vi "CSTK_Button_Icon_Init.vi"(3 "Container State":T20 caption="容器状态", 4 "Previous State":variant caption="前期状态", 5 "Previous Version":T19 caption="前期版本") -> (2 "Current State":T1={"ButtonSize"={"False"={"Width"=0, "Height"=0}, "True"={"Width"=0, "Height"=0}, "True to False"={"Width"=0, "Height"=0}, "False to True"={"Width"=0, "Height"=0}, "Hover in False"={"Width"=0, "Height"=0}, "Hover in True"={"Width"=0, "Height"=0}}, "Logo Image"={"False"={"image type"=0, "image depth"=0, "image"=[], "mask"=[], "colors"=[], "Rectangle"={"left"=0, "top"=0, "right"=0, "bottom"=0}}, "True"={"image type"=0, "image depth"=0, "image"=[], "mask"=[], "colors"=[], "Rectangle"={"left"=0, "top"=0, "right"=0, "bottom"=0}}, "True to False"={"image type"=0, "image depth"=0, "image"=[], "mask"=[], "colors"=[], "Rectangle"={"left"=0, "top"=0, "right"=0, "bottom"=0}}, "False to True"={"image type"=0, "image depth"=0, "image"=[], "mask"=[], "colors"=[], "Rectangle"={"left"=0, "top"=0, "right"=0, "bottom"=0}}, "Hover in False"={"image type"=0, "image depth"=0, "image"=[], "mask"=[], "colors"=[], "Rectangle"={"left"=0, "top"=0, "right"=0, "bottom"=0}}, "Hover in True"={"image type"=0, "image depth"=0, "image"=[], "mask"=[], "colors"=[], "Rectangle"={"left"=0, "top"=0, "right"=0, "bottom"=0}}}, "Logo Properties"={"False"={"Display Logo?"=FALSE, "Horizontal Offset"=0}, "True"={"Display Logo?"=FALSE, "Horizontal Offset"=0}, "True to False"={"Display Logo?"=FALSE, "Horizontal Offset"=0}, "False to True"={"Display Logo?"=FALSE, "Horizontal Offset"=0}, "Hover in False"={"Display Logo?"=FALSE, "Horizontal Offset"=0}, "Hover in True"={"Display Logo?"=FALSE, "Horizontal Offset"=0}}, "Text String"={"False"="", "True"="", "True to False"="", "False to True"="", "Hover in False"="", "Hover in True"=""}, "Text Properties"={"False"={"Display Text?"=FALSE, "Text Color"=0, "Horizontal Offset"=0, "Font Style"={"Font Name"="", "Size"=0, "Strikeout?"=FALSE, "Italic?"=FALSE, "Underline?"=FALSE, "Outline?"=FALSE, "Shadow?"=FALSE, "Bold?"=FALSE}}, "True"={"Display Text?"=FALSE, "Text Color"=0, "Horizontal Offset"=0, "Font Style"={"Font Name"="", "Size"=0, "Strikeout?"=FALSE, "Italic?"=FALSE, "Underline?"=FALSE, "Outline?"=FALSE, "Shadow?"=FALSE, "Bold?"=FALSE}}, "True to False"={"Display Text?"=FALSE, "Text Color"=0, "Horizontal Offset"=0, "Font Style"={"Font Name"="", "Size"=0, "Strikeout?"=FALSE, "Italic?"=FALSE, "Underline?"=FALSE, "Outline?"=FALSE, "Shadow?"=FALSE, "Bold?"=FALSE}}, "False to True"={"Display Text?"=FALSE, "Text Color"=0, "Horizontal Offset"=0, "Font Style"={"Font Name"="", "Size"=0, "Strikeout?"=FALSE, "Italic?"=FALSE, "Underline?"=FALSE, "Outline?"=FALSE, "Shadow?"=FALSE, "Bold?"=FALSE}}, "Hover in False"={"Display Text?"=FALSE, "Text Color"=0, "Horizontal Offset"=0, "Font Style"={"Font Name"="", "Size"=0, "Strikeout?"=FALSE, "Italic?"=FALSE, "Underline?"=FALSE, "Outline?"=FALSE, "Shadow?"=FALSE, "Bold?"=FALSE}}, "Hover in True"={"Display Text?"=FALSE, "Text Color"=0, "Horizontal Offset"=0, "Font Style"={"Font Name"="", "Size"=0, "Strikeout?"=FALSE, "Italic?"=FALSE, "Underline?"=FALSE, "Outline?"=FALSE, "Shadow?"=FALSE, "Bold?"=FALSE}}}, "BG Color"={"False"=0, "True"=0, "True to False"=0, "False to True"=0, "Hover in False"=0, "Hover in True"=0}, "Border Color"={"False"=0, "True"=0, "True to False"=0, "False to True"=0, "Hover in False"=0, "Hover in True"=0}, "Border Properties"={"False"={"Radius"=0, "Border Style"={"Width"=3, "Style"=enum."Solid"}}, "True"={"Radius"=0, "Border Style"={"Width"=3, "Style"=enum."Solid"}}, "True to False"={"Radius"=0, "Border Style"={"Width"=3, "Style"=enum."Solid"}}, "False to True"={"Radius"=0, "Border Style"={"Width"=3, "Style"=enum."Solid"}}, "Hover in False"={"Radius"=0, "Border Style"={"Width"=3, "Style"=enum."Solid"}}, "Hover in True"={"Radius"=0, "Border Style"={"Width"=3, "Style"=enum."Solid"}}}, "Current BG Image"={"False"=bytes[0], "True"=bytes[0], "True to False"=bytes[0], "False to True"=bytes[0], "Hover in False"=bytes[0], "Hover in True"=bytes[0]}, "DrawAreaSize"={"False"={"Width"=0, "Height"=0}, "True"={"Width"=0, "Height"=0}, "True to False"={"Width"=0, "Height"=0}, "False to True"={"Width"=0, "Height"=0}, "Hover in False"={"Width"=0, "Height"=0}, "Hover in True"={"Width"=0, "Height"=0}}, "Text String Offset"={"False"=0, "True"=0, "True to False"=0, "False to True"=0, "Hover in False"=0, "Hover in True"=0}} caption="当前状态")   [LabVIEW 2015, in "CSTK_Button_Icon.xctl"]
uses:
  CSTK_Button_Icon.xctl
  CSTK_Button_Icon_Status.ctl
  Private/TypeDefinitions/_CSTK_Button_Icon_ButtonSize.ctl
  <vilib>/Utility/miscctls.llb/LVBoundsTypeDef.ctl
  Private/TypeDefinitions/_CSTK_Button_Icon_LogoImage.ctl
  <vilib>/picture/picture.llb/imagedata.ctl
  Private/TypeDefinitions/_CSTK_Button_Icon_LogoProperties.ctl
  Private/TypeDefinitions/_CSTK_Button_Icon_LogoProperties_Data.ctl
  Private/TypeDefinitions/_CSTK_Button_Icon_TextString.ctl
  Private/TypeDefinitions/_CSTK_Button_Icon_TextProperties.ctl
  Private/TypeDefinitions/_CSTK_Button_Icon_TextProperties_Data.ctl
  Private/TypeDefinitions/_CSTK_Button_Icon_TextProperties_FontStyle.ctl
  Private/TypeDefinitions/_CSTK_Button_Icon_BGColor.ctl
  Private/TypeDefinitions/_CSTK_Button_Icon_BorderColor.ctl
  Private/TypeDefinitions/_CSTK_Button_Icon_BorderProperties.ctl
  Private/TypeDefinitions/_CSTK_Button_Icon_BorderProperties_Data.ctl
  Private/TypeDefinitions/_CSTK_Button_Icon_CurrentBGImage.ctl
  Private/TypeDefinitions/_CSTK_Button_Icon_DrawAreaSize.ctl
  Private/TypeDefinitions/_CSTK_Button_Icon_TextStartOffset.ctl
  <vilib>/_xctls/Container State.ctl
  <vilib>/_xctls/Version.ctl
  <vilib>/_xctls/XControlSupport.lvlib
panel:
  in  "Default Indicator State":T1={"ButtonSize"={"False"={"Width"=120, "Height"=36}, "True"={"Width"=120, "Height"=36}, "True to False"={"Width"=120, "Height"=36}, "False to True"={"Width"=120, "Height"=36}, "Hover in False"={"Width"=120, "Height"=36}, "Hover in True"={"Width"=120, "Height"=36}}, "Logo Image"={"False"={"image type"=0, "image depth"=32, "image"=array[2304 elements], "mask"=[0, 0, 0, 0, 0, 0, 0, 0, 0, 0, 0, 0, 0, 0, 0, 0, 0, 0, 0, 0, 0, 0, 12, 0, 0, 0, 28, 0, 0, 0, 60, 0, 0, 0, 120, 0, 0, 0, 240, 0, 48, 1, 224, 0, 56, 3, 192, 0, 28, 7, 128, 0, 14, 15, 0, 0, 7, 30, 0, 0, 3, 188, 0, 0, 1, 248, 0, 0, 0, 240, 0, 0, 0, 96, 0, 0, 0, 0, 0, 0, 0, 0, 0, 0, 0, 0, 0, 0, 0, 0, 0, 0, 0, 0, 0, 0], "colors"=[], "Rectangle"={"left"=0, "top"=0, "right"=24, "bottom"=24}}, "True"={"image type"=0, "image depth"=32, "image"=array[2304 elements], "mask"=[0, 0, 0, 0, 0, 0, 0, 0, 0, 0, 0, 0, 0, 0, 0, 0, 0, 0, 0, 0, 0, 0, 12, 0, 0, 0, 28, 0, 0, 0, 60, 0, 0, 0, 120, 0, 0, 0, 240, 0, 48, 1, 224, 0, 56, 3, 192, 0, 28, 7, 128, 0, 14, 15, 0, 0, 7, 30, 0, 0, 3, 188, 0, 0, 1, 248, 0, 0, 0, 240, 0, 0, 0, 96, 0, 0, 0, 0, 0, 0, 0, 0, 0, 0, 0, 0, 0, 0, 0, 0, 0, 0, 0, 0, 0, 0], "colors"=[], "Rectangle"={"left"=0, "top"=0, "right"=24, "bottom"=24}}, "True to False"={"image type"=0, "image depth"=32, "image"=array[2304 elements], "mask"=[0, 0, 0, 0, 0, 0, 0, 0, 0, 0, 0, 0, 0, 0, 0, 0, 0, 0, 0, 0, 0, 0, 12, 0, 0, 0, 28, 0, 0, 0, 60, 0, 0, 0, 120, 0, 0, 0, 240, 0, 48, 1, 224, 0, 56, 3, 192, 0, 28, 7, 128, 0, 14, 15, 0, 0, 7, 30, 0, 0, 3, 188, 0, 0, 1, 248, 0, 0, 0, 240, 0, 0, 0, 96, 0, 0, 0, 0, 0, 0, 0, 0, 0, 0, 0, 0, 0, 0, 0, 0, 0, 0, 0, 0, 0, 0], "colors"=[], "Rectangle"={"left"=0, "top"=0, "right"=24, "bottom"=24}}, "False to True"={"image type"=0, "image depth"=32, "image"=array[2304 elements], "mask"=[0, 0, 0, 0, 0, 0, 0, 0, 0, 0, 0, 0, 0, 0, 0, 0, 0, 0, 0, 0, 0, 0, 12, 0, 0, 0, 28, 0, 0, 0, 60, 0, 0, 0, 120, 0, 0, 0, 240, 0, 48, 1, 224, 0, 56, 3, 192, 0, 28, 7, 128, 0, 14, 15, 0, 0, 7, 30, 0, 0, 3, 188, 0, 0, 1, 248, 0, 0, 0, 240, 0, 0, 0, 96, 0, 0, 0, 0, 0, 0, 0, 0, 0, 0, 0, 0, 0, 0, 0, 0, 0, 0, 0, 0, 0, 0], "colors"=[], "Rectangle"={"left"=0, "top"=0, "right"=24, "bottom"=24}}, "Hover in False"={"image type"=0, "image depth"=32, "image"=array[2304 elements], "mask"=[0, 0, 0, 0, 0, 0, 0, 0, 0, 0, 0, 0, 0, 0, 0, 0, 0, 0, 0, 0, 0, 0, 12, 0, 0, 0, 28, 0, 0, 0, 60, 0, 0, 0, 120, 0, 0, 0, 240, 0, 48, 1, 224, 0, 56, 3, 192, 0, 28, 7, 128, 0, 14, 15, 0, 0, 7, 30, 0, 0, 3, 188, 0, 0, 1, 248, 0, 0, 0, 240, 0, 0, 0, 96, 0, 0, 0, 0, 0, 0, 0, 0, 0, 0, 0, 0, 0, 0, 0, 0, 0, 0, 0, 0, 0, 0], "colors"=[], "Rectangle"={"left"=0, "top"=0, "right"=24, "bottom"=24}}, "Hover in True"={"image type"=0, "image depth"=32, "image"=array[2304 elements], "mask"=[0, 0, 0, 0, 0, 0, 0, 0, 0, 0, 0, 0, 0, 0, 0, 0, 0, 0, 0, 0, 0, 0, 12, 0, 0, 0, 28, 0, 0, 0, 60, 0, 0, 0, 120, 0, 0, 0, 240, 0, 48, 1, 224, 0, 56, 3, 192, 0, 28, 7, 128, 0, 14, 15, 0, 0, 7, 30, 0, 0, 3, 188, 0, 0, 1, 248, 0, 0, 0, 240, 0, 0, 0, 96, 0, 0, 0, 0, 0, 0, 0, 0, 0, 0, 0, 0, 0, 0, 0, 0, 0, 0, 0, 0, 0, 0], "colors"=[], "Rectangle"={"left"=0, "top"=0, "right"=24, "bottom"=24}}}, "Logo Properties"={"False"={"Display Logo?"=TRUE, "Horizontal Offset"=0}, "True"={"Display Logo?"=TRUE, "Horizontal Offset"=0}, "True to False"={"Display Logo?"=TRUE, "Horizontal Offset"=0}, "False to True"={"Display Logo?"=TRUE, "Horizontal Offset"=0}, "Hover in False"={"Display Logo?"=TRUE, "Horizontal Offset"=0}, "Hover in True"={"Display Logo?"=TRUE, "Horizontal Offset"=0}}, "Text String"={"False"="Fasle", "True"="True", "True to False"="False", "False to True"="True", "Hover in False"="Fasle", "Hover in True"="True"}, "Text Properties"={"False"={"Display Text?"=TRUE, "Text Color"=0, "Horizontal Offset"=0, "Font Style"={"Font Name"="", "Size"=17, "Strikeout?"=FALSE, "Italic?"=FALSE, "Underline?"=FALSE, "Outline?"=FALSE, "Shadow?"=FALSE, "Bold?"=FALSE}}, "True"={"Display Text?"=TRUE, "Text Color"=0, "Horizontal Offset"=0, "Font Style"={"Font Name"="", "Size"=17, "Strikeout?"=FALSE, "Italic?"=FALSE, "Underline?"=FALSE, "Outline?"=FALSE, "Shadow?"=FALSE, "Bold?"=FALSE}}, "True to False"={"Display Text?"=TRUE, "Text Color"=0, "Horizontal Offset"=0, "Font Style"={"Font Name"="", "Size"=17, "Strikeout?"=FALSE, "Italic?"=FALSE, "Underline?"=FALSE, "Outline?"=FALSE, "Shadow?"=FALSE, "Bold?"=FALSE}}, "False to True"={"Display Text?"=TRUE, "Text Color"=0, "Horizontal Offset"=0, "Font Style"={"Font Name"="", "Size"=17, "Strikeout?"=FALSE, "Italic?"=FALSE, "Underline?"=FALSE, "Outline?"=FALSE, "Shadow?"=FALSE, "Bold?"=FALSE}}, "Hover in False"={"Display Text?"=TRUE, "Text Color"=0, "Horizontal Offset"=0, "Font Style"={"Font Name"="", "Size"=17, "Strikeout?"=FALSE, "Italic?"=FALSE, "Underline?"=FALSE, "Outline?"=FALSE, "Shadow?"=FALSE, "Bold?"=FALSE}}, "Hover in True"={"Display Text?"=TRUE, "Text Color"=0, "Horizontal Offset"=0, "Font Style"={"Font Name"="", "Size"=17, "Strikeout?"=FALSE, "Italic?"=FALSE, "Underline?"=FALSE, "Outline?"=FALSE, "Shadow?"=FALSE, "Bold?"=FALSE}}}, "BG Color"={"False"=14869218, "True"=16744576, "True to False"=14869218, "False to True"=16744576, "Hover in False"=14869218, "Hover in True"=16744576}, "Border Color"={"False"=11251123, "True"=11251123, "True to False"=11251123, "False to True"=11251123, "Hover in False"=11251123, "Hover in True"=11251123}, "Border Properties"={"False"={"Radius"=10, "Border Style"={"Width"=3, "Style"=enum."Solid"}}, "True"={"Radius"=10, "Border Style"={"Width"=3, "Style"=enum."Solid"}}, "True to False"={"Radius"=10, "Border Style"={"Width"=3, "Style"=enum."Solid"}}, "False to True"={"Radius"=10, "Border Style"={"Width"=3, "Style"=enum."Solid"}}, "Hover in False"={"Radius"=10, "Border Style"={"Width"=3, "Style"=enum."Solid"}}, "Hover in True"={"Radius"=10, "Border Style"={"Width"=3, "Style"=enum."Solid"}}}, "Current BG Image"={"False"=bytes[0], "True"=bytes[0], "True to False"=bytes[0], "False to True"=bytes[0], "Hover in False"=bytes[0], "Hover in True"=bytes[0]}, "DrawAreaSize"={"False"={"Width"=0, "Height"=0}, "True"={"Width"=0, "Height"=0}, "True to False"={"Width"=0, "Height"=0}, "False to True"={"Width"=0, "Height"=0}, "Hover in False"={"Width"=0, "Height"=0}, "Hover in True"={"Width"=0, "Height"=0}}, "Text String Offset"={"False"=0, "True"=0, "True to False"=0, "False to True"=0, "Hover in False"=0, "Hover in True"=0}} caption="默认显示控件状态"
  in  "Default Control State":T1={"ButtonSize"={"False"={"Width"=120, "Height"=36}, "True"={"Width"=120, "Height"=36}, "True to False"={"Width"=120, "Height"=36}, "False to True"={"Width"=120, "Height"=36}, "Hover in False"={"Width"=120, "Height"=36}, "Hover in True"={"Width"=120, "Height"=36}}, "Logo Image"={"False"={"image type"=0, "image depth"=32, "image"=array[2304 elements], "mask"=[0, 0, 0, 0, 0, 0, 0, 0, 0, 0, 0, 0, 0, 0, 0, 0, 0, 0, 0, 0, 0, 0, 12, 0, 0, 0, 28, 0, 0, 0, 60, 0, 0, 0, 120, 0, 0, 0, 240, 0, 48, 1, 224, 0, 56, 3, 192, 0, 28, 7, 128, 0, 14, 15, 0, 0, 7, 30, 0, 0, 3, 188, 0, 0, 1, 248, 0, 0, 0, 240, 0, 0, 0, 96, 0, 0, 0, 0, 0, 0, 0, 0, 0, 0, 0, 0, 0, 0, 0, 0, 0, 0, 0, 0, 0, 0], "colors"=[], "Rectangle"={"left"=0, "top"=0, "right"=24, "bottom"=24}}, "True"={"image type"=0, "image depth"=32, "image"=array[2304 elements], "mask"=[0, 0, 0, 0, 0, 0, 0, 0, 0, 0, 0, 0, 0, 0, 0, 0, 0, 0, 0, 0, 0, 0, 12, 0, 0, 0, 28, 0, 0, 0, 60, 0, 0, 0, 120, 0, 0, 0, 240, 0, 48, 1, 224, 0, 56, 3, 192, 0, 28, 7, 128, 0, 14, 15, 0, 0, 7, 30, 0, 0, 3, 188, 0, 0, 1, 248, 0, 0, 0, 240, 0, 0, 0, 96, 0, 0, 0, 0, 0, 0, 0, 0, 0, 0, 0, 0, 0, 0, 0, 0, 0, 0, 0, 0, 0, 0], "colors"=[], "Rectangle"={"left"=0, "top"=0, "right"=24, "bottom"=24}}, "True to False"={"image type"=0, "image depth"=32, "image"=array[2304 elements], "mask"=[0, 0, 0, 0, 0, 0, 0, 0, 0, 0, 0, 0, 0, 0, 0, 0, 0, 0, 0, 0, 0, 0, 12, 0, 0, 0, 28, 0, 0, 0, 60, 0, 0, 0, 120, 0, 0, 0, 240, 0, 48, 1, 224, 0, 56, 3, 192, 0, 28, 7, 128, 0, 14, 15, 0, 0, 7, 30, 0, 0, 3, 188, 0, 0, 1, 248, 0, 0, 0, 240, 0, 0, 0, 96, 0, 0, 0, 0, 0, 0, 0, 0, 0, 0, 0, 0, 0, 0, 0, 0, 0, 0, 0, 0, 0, 0], "colors"=[], "Rectangle"={"left"=0, "top"=0, "right"=24, "bottom"=24}}, "False to True"={"image type"=0, "image depth"=32, "image"=array[2304 elements], "mask"=[0, 0, 0, 0, 0, 0, 0, 0, 0, 0, 0, 0, 0, 0, 0, 0, 0, 0, 0, 0, 0, 0, 12, 0, 0, 0, 28, 0, 0, 0, 60, 0, 0, 0, 120, 0, 0, 0, 240, 0, 48, 1, 224, 0, 56, 3, 192, 0, 28, 7, 128, 0, 14, 15, 0, 0, 7, 30, 0, 0, 3, 188, 0, 0, 1, 248, 0, 0, 0, 240, 0, 0, 0, 96, 0, 0, 0, 0, 0, 0, 0, 0, 0, 0, 0, 0, 0, 0, 0, 0, 0, 0, 0, 0, 0, 0], "colors"=[], "Rectangle"={"left"=0, "top"=0, "right"=24, "bottom"=24}}, "Hover in False"={"image type"=0, "image depth"=32, "image"=array[2304 elements], "mask"=[0, 0, 0, 0, 0, 0, 0, 0, 0, 0, 0, 0, 0, 0, 0, 0, 0, 0, 0, 0, 0, 0, 12, 0, 0, 0, 28, 0, 0, 0, 60, 0, 0, 0, 120, 0, 0, 0, 240, 0, 48, 1, 224, 0, 56, 3, 192, 0, 28, 7, 128, 0, 14, 15, 0, 0, 7, 30, 0, 0, 3, 188, 0, 0, 1, 248, 0, 0, 0, 240, 0, 0, 0, 96, 0, 0, 0, 0, 0, 0, 0, 0, 0, 0, 0, 0, 0, 0, 0, 0, 0, 0, 0, 0, 0, 0], "colors"=[], "Rectangle"={"left"=0, "top"=0, "right"=24, "bottom"=24}}, "Hover in True"={"image type"=0, "image depth"=32, "image"=array[2304 elements], "mask"=[0, 0, 0, 0, 0, 0, 0, 0, 0, 0, 0, 0, 0, 0, 0, 0, 0, 0, 0, 0, 0, 0, 12, 0, 0, 0, 28, 0, 0, 0, 60, 0, 0, 0, 120, 0, 0, 0, 240, 0, 48, 1, 224, 0, 56, 3, 192, 0, 28, 7, 128, 0, 14, 15, 0, 0, 7, 30, 0, 0, 3, 188, 0, 0, 1, 248, 0, 0, 0, 240, 0, 0, 0, 96, 0, 0, 0, 0, 0, 0, 0, 0, 0, 0, 0, 0, 0, 0, 0, 0, 0, 0, 0, 0, 0, 0], "colors"=[], "Rectangle"={"left"=0, "top"=0, "right"=24, "bottom"=24}}}, "Logo Properties"={"False"={"Display Logo?"=TRUE, "Horizontal Offset"=0}, "True"={"Display Logo?"=TRUE, "Horizontal Offset"=0}, "True to False"={"Display Logo?"=TRUE, "Horizontal Offset"=0}, "False to True"={"Display Logo?"=TRUE, "Horizontal Offset"=0}, "Hover in False"={"Display Logo?"=TRUE, "Horizontal Offset"=0}, "Hover in True"={"Display Logo?"=TRUE, "Horizontal Offset"=0}}, "Text String"={"False"="OK", "True"="OK", "True to False"="OK", "False to True"="OK", "Hover in False"="OK", "Hover in True"="OK"}, "Text Properties"={"False"={"Display Text?"=TRUE, "Text Color"=0, "Horizontal Offset"=0, "Font Style"={"Font Name"="", "Size"=17, "Strikeout?"=FALSE, "Italic?"=FALSE, "Underline?"=FALSE, "Outline?"=FALSE, "Shadow?"=FALSE, "Bold?"=FALSE}}, "True"={"Display Text?"=TRUE, "Text Color"=0, "Horizontal Offset"=0, "Font Style"={"Font Name"="", "Size"=17, "Strikeout?"=FALSE, "Italic?"=FALSE, "Underline?"=FALSE, "Outline?"=FALSE, "Shadow?"=FALSE, "Bold?"=FALSE}}, "True to False"={"Display Text?"=TRUE, "Text Color"=0, "Horizontal Offset"=0, "Font Style"={"Font Name"="", "Size"=17, "Strikeout?"=FALSE, "Italic?"=FALSE, "Underline?"=FALSE, "Outline?"=FALSE, "Shadow?"=FALSE, "Bold?"=FALSE}}, "False to True"={"Display Text?"=TRUE, "Text Color"=0, "Horizontal Offset"=0, "Font Style"={"Font Name"="", "Size"=17, "Strikeout?"=FALSE, "Italic?"=FALSE, "Underline?"=FALSE, "Outline?"=FALSE, "Shadow?"=FALSE, "Bold?"=FALSE}}, "Hover in False"={"Display Text?"=TRUE, "Text Color"=0, "Horizontal Offset"=0, "Font Style"={"Font Name"="", "Size"=17, "Strikeout?"=FALSE, "Italic?"=FALSE, "Underline?"=FALSE, "Outline?"=FALSE, "Shadow?"=FALSE, "Bold?"=FALSE}}, "Hover in True"={"Display Text?"=TRUE, "Text Color"=0, "Horizontal Offset"=0, "Font Style"={"Font Name"="", "Size"=17, "Strikeout?"=FALSE, "Italic?"=FALSE, "Underline?"=FALSE, "Outline?"=FALSE, "Shadow?"=FALSE, "Bold?"=FALSE}}}, "BG Color"={"False"=12632319, "True"=16761024, "True to False"=8421631, "False to True"=16744576, "Hover in False"=10263807, "Hover in True"=16751772}, "Border Color"={"False"=11251123, "True"=11251123, "True to False"=11251123, "False to True"=11251123, "Hover in False"=11251123, "Hover in True"=11251123}, "Border Properties"={"False"={"Radius"=10, "Border Style"={"Width"=3, "Style"=enum."Solid"}}, "True"={"Radius"=10, "Border Style"={"Width"=3, "Style"=enum."Solid"}}, "True to False"={"Radius"=10, "Border Style"={"Width"=3, "Style"=enum."Solid"}}, "False to True"={"Radius"=10, "Border Style"={"Width"=3, "Style"=enum."Solid"}}, "Hover in False"={"Radius"=10, "Border Style"={"Width"=3, "Style"=enum."Solid"}}, "Hover in True"={"Radius"=10, "Border Style"={"Width"=3, "Style"=enum."Solid"}}}, "Current BG Image"={"False"=bytes[0], "True"=bytes[0], "True to False"=bytes[0], "False to True"=bytes[0], "Hover in False"=bytes[0], "Hover in True"=bytes[0]}, "DrawAreaSize"={"False"={"Width"=0, "Height"=0}, "True"={"Width"=0, "Height"=0}, "True to False"={"Width"=0, "Height"=0}, "False to True"={"Width"=0, "Height"=0}, "Hover in False"={"Width"=0, "Height"=0}, "Hover in True"={"Width"=0, "Height"=0}}, "Text String Offset"={"False"=0, "True"=0, "True to False"=0, "False to True"=0, "Hover in False"=0, "Hover in True"=0}} caption="默认输入控件状态"
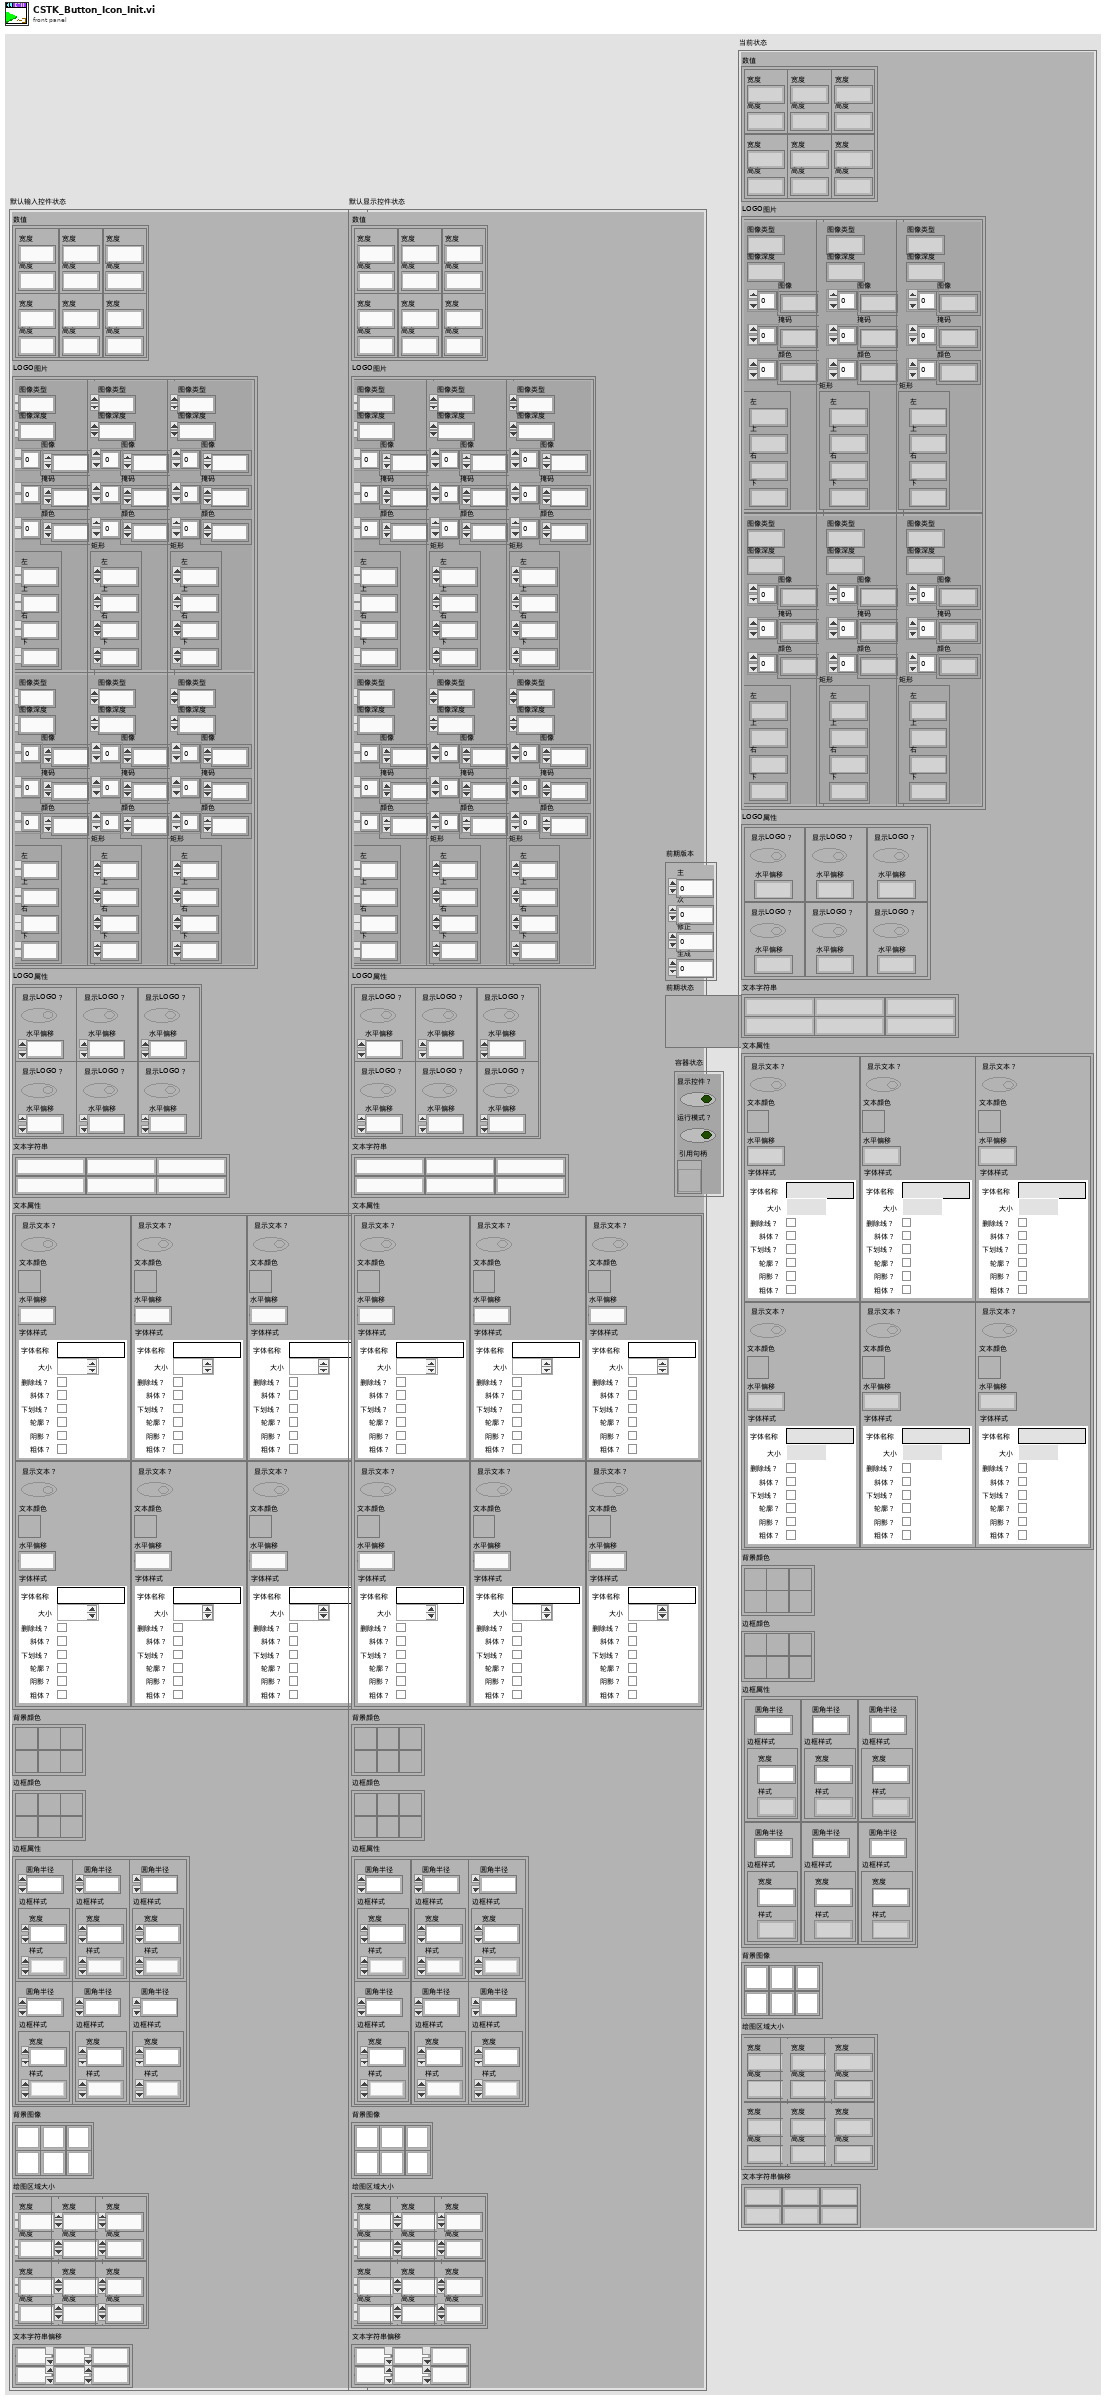
[diagram p1: front panel]
types:
  T1 = typedef "CSTK_Button_Icon.xctl/CSTK_Button_Icon_Status.ctl" = cluster{"ButtonSize":T2, "Logo Image":T4, "Logo Properties":T6, "Text String":T8, "Text Properties":T9, "BG Color":T12, "Border Color":T13, "Border Properties":T14, "Current BG Image":T16, "DrawAreaSize":T17, "Text String Offset":T18}
  T2 = typedef "CSTK_Button_Icon.xctl/_CSTK_Button_Icon_ButtonSize.ctl" = cluster{"False":T3, "True":T3, "True to False":T3, "False to True":T3, "Hover in False":T3, "Hover in True":T3}
  T3 = typedef "LVBoundsTypeDef.ctl" = cluster{"Width":u32, "Height":u32}
  T4 = typedef "CSTK_Button_Icon.xctl/_CSTK_Button_Icon_LogoImage.ctl" = cluster{"False":T5, "True":T5, "True to False":T5, "False to True":T5, "Hover in False":T5, "Hover in True":T5}
  T5 = typedef "imagedata.ctl" = cluster{"image type":i32, "image depth":i32, "image":u8[], "mask":u8[], "colors":u32[], "Rectangle":cluster{"left":i16, "top":i16, "right":i16, "bottom":i16}}
  T6 = typedef "CSTK_Button_Icon.xctl/_CSTK_Button_Icon_LogoProperties.ctl" = cluster{"False":T7, "True":T7, "True to False":T7, "False to True":T7, "Hover in False":T7, "Hover in True":T7}
  T7 = typedef "CSTK_Button_Icon.xctl/_CSTK_Button_Icon_LogoProperties_Data.ctl" = cluster{"Display Logo?":bool, "Horizontal Offset":i16}
  T8 = typedef "CSTK_Button_Icon.xctl/_CSTK_Button_Icon_TextString.ctl" = cluster{"False":string, "True":string, "True to False":string, "False to True":string, "Hover in False":string, "Hover in True":string}
  T9 = typedef "CSTK_Button_Icon.xctl/_CSTK_Button_Icon_TextProperties.ctl" = cluster{"False":T10, "True":T10, "True to False":T10, "False to True":T10, "Hover in False":T10, "Hover in True":T10}
  T10 = typedef "CSTK_Button_Icon.xctl/_CSTK_Button_Icon_TextProperties_Data.ctl" = cluster{"Display Text?":bool, "Text Color":u32, "Horizontal Offset":i16, "Font Style":T11}
  T11 = typedef "CSTK_Button_Icon.xctl/_CSTK_Button_Icon_TextProperties_FontStyle.ctl" = cluster{"Font Name":string, "Size":i16, "Strikeout?":bool, "Italic?":bool, "Underline?":bool, "Outline?":bool, "Shadow?":bool, "Bold?":bool}
  T12 = typedef "CSTK_Button_Icon.xctl/_CSTK_Button_Icon_BGColor.ctl" = cluster{"False":u32, "True":u32, "True to False":u32, "False to True":u32, "Hover in False":u32, "Hover in True":u32}
  T13 = typedef "CSTK_Button_Icon.xctl/_CSTK_Button_Icon_BorderColor.ctl" = cluster{"False":u32, "True":u32, "True to False":u32, "False to True":u32, "Hover in False":u32, "Hover in True":u32}
  T14 = typedef "CSTK_Button_Icon.xctl/_CSTK_Button_Icon_BorderProperties.ctl" = cluster{"False":T15, "True":T15, "True to False":T15, "False to True":T15, "Hover in False":T15, "Hover in True":T15}
  T15 = typedef "CSTK_Button_Icon.xctl/_CSTK_Button_Icon_BorderProperties_Data.ctl" = cluster{"Radius":i16, "Border Style":cluster{"Width":u16, "Style":enum32{"Solid", "Dash", "Dot", "DashDot", "DashDotDot"}}}
  T16 = typedef "CSTK_Button_Icon.xctl/_CSTK_Button_Icon_CurrentBGImage.ctl" = cluster{"False":picture, "True":picture, "True to False":picture, "False to True":picture, "Hover in False":picture, "Hover in True":picture}
  T17 = typedef "CSTK_Button_Icon.xctl/_CSTK_Button_Icon_DrawAreaSize.ctl" = cluster{"False":T3, "True":T3, "True to False":T3, "False to True":T3, "Hover in False":T3, "Hover in True":T3}
  T18 = typedef "CSTK_Button_Icon.xctl/_CSTK_Button_Icon_TextStartOffset.ctl" = cluster{"False":i32, "True":i32, "True to False":i32, "False to True":i32, "Hover in False":i32, "Hover in True":i32}
  T19 = typedef "XControlSupport.lvlib/Version.ctl" = cluster{"Major":u16, "Minor":u16, "Fix":u16, "Build":u16}
  T20 = typedef "XControlSupport.lvlib/Container State.ctl" = cluster{"Indicator?":bool, "Run Mode?":bool, " Refnum":refnum<vi>}
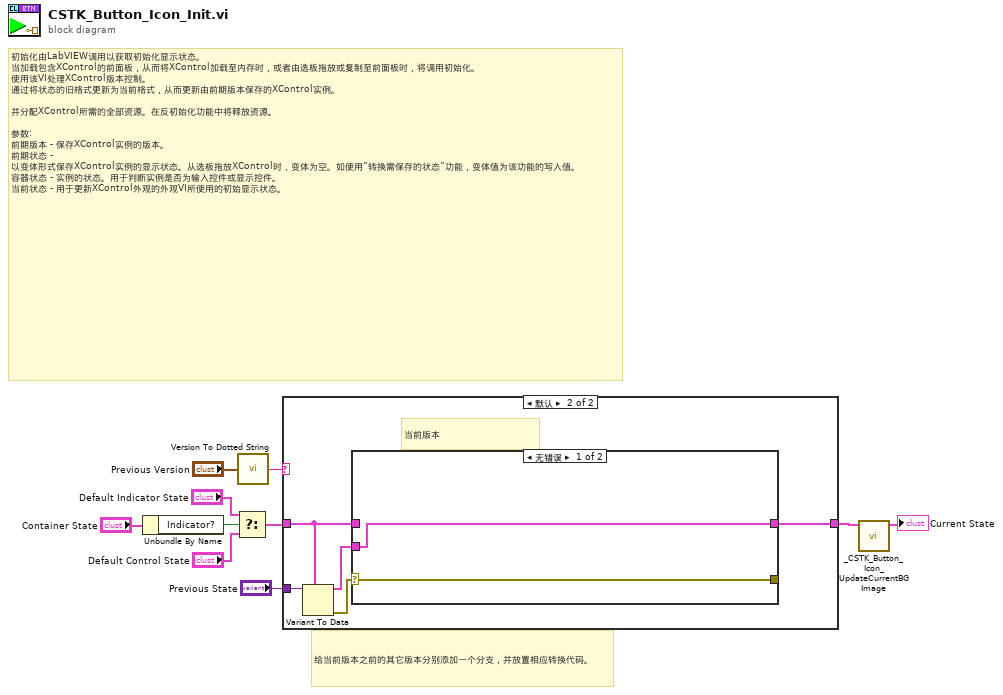
[diagram p0: block diagram]
diagram:
  # "给当前版本之前的其它版本分别添加一个分支，并放置相应转换代码。"
  # "初始化由LabVIEW调用以获取初始化显示状态。\n当加载包含XControl的前面板，从而将XControl加载至内存时，或者由选板拖放或复制至前面板时，将调用初始化。\n使用该VI处理XControl版本控制。\n通过将状态的旧格式更新为当前格式，从而更新由前期版本保存的XControl实例。\n\n并分配XControl所需的全部资源。在反初始化功能中将释放资源。\n\n参数: \n前期版本 - 保存XControl实例的版本。\n前期状态 - 以变体形式保存XControl实例的显示状态。从选板拖放XControl时，变体为空。如使用“转换需保存的状态”功能，变体值为该功能的写入值。\n容器状态 - 实例的状态。用于判断实例是否为输入控件或显示控件。\n当前状态 - 用于更新XControl外观的外观VI所使用的初始显示状态。"
  n1 = Unbundle By Name("Container State") -> ("Indicator?"=w7:bool)
  n2 = Select(t="Default Indicator State", s=w7, f="Default Control State") -> (s? t:f=w6:T1)
  n3 = call <vilib>:"Version To Dotted String.vi"("Version"="Previous Version") -> ("String Version"=w4:string)
  n4 = case shown="默认" w4 {
    tunnel: "Previous State" -> [_ w16]
    tunnel: [w11 w12] -> w2
    tunnel: w6 -> [w11 w13]
    frame "0.0.0.0" {
      # "已创建，并使用默认状态"
    }
    frame Default {
      # "当前版本"
      n5 = Variant To Data(type=w13, Variant=w16) -> (data=w14:T1, error out=w15:errorcluster)  [unwired: 1 in]
      n6 = case shown="无错误" w15 {
        selector: w15 -> [w18 w19]
        tunnel: w14 -> [w17 _]
        tunnel: [w17 w20] -> w12
        tunnel: w13 -> [_ w20]
        tunnel: [w18 w19] -> _
        frame No Error {
        }
        frame Error {
          # "转换前期保存状态时\n发生错误。使用默认。"
        }
      }
    }
  }
  n7 = call "_CSTK_Button_Icon_UpdateCurrentBGImage.vi"("State in"=w2) -> ("State out"=→"Current State":T1)  [unwired: 10 in]
